vi "WPI_CameraWhiteBalanceConstants.vi"() -> (3 "Color Temps (K)":dbl[](array[numeric]))   [LabVIEW 2017]
doc: "Returns the Kelvin temperatures that correspond to the enum used by Axis."
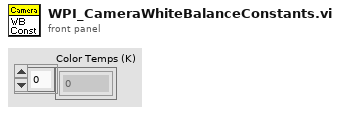
[diagram p1: front panel]
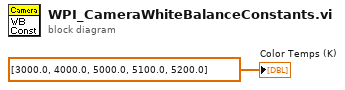
[diagram p0: block diagram]
diagram:
  "Color Temps (K)" <- dbl[] [3000.0, 4000.0, 5000.0, 5100.0, 5200.0]
